vi "Reduce Funds.vi"(6 "wait for reply (T)":bool=TRUE, 8 "error in (no error)":errorcluster, 10 "Reduce Funds":i32) -> (0 "error out":errorcluster, 1 "timed out?":bool, 2 "Sucessful":bool, 3 "Remaining Balance":u32, 5 "Reply Payload":T1)   [LabVIEW 2020, in "Money.lvlib"]
doc: "Reduce Funds\n_____\nCreated using Delacor QMH Event Scripter 4.2.1.88."
uses:
  Money.lvlib
  Reduce Funds (Reply Payload)--cluster.ctl
  Reduce Funds Argument--cluster.ctl
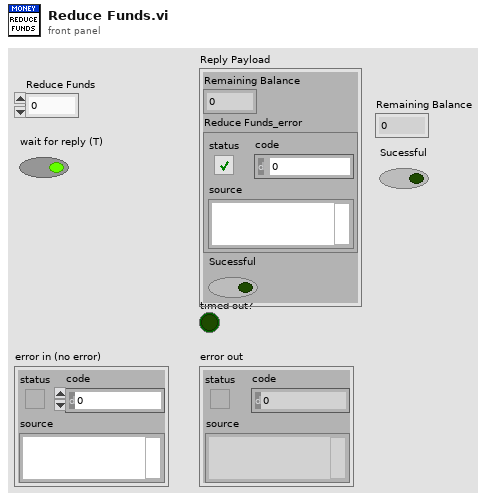
[diagram p1: front panel]
types:
  T1 = typedef "Money.lvlib/Reduce Funds (Reply Payload)--cluster.ctl" = cluster{"Remaining Balance":u32, "Reduce Funds_error":errorcluster, "Sucessful":bool}
  T2 = typedef "Money.lvlib/Reduce Funds Argument--cluster.ctl" = cluster{"Reduce Funds":i32, "Wait Notifier":refnum<notifier>, "wait for reply":bool}
  T3 = typedef "Money.lvlib/Request Events--cluster.ctl" = cluster{"Stop Module":refnum<user-event>, "Show Panel":refnum<user-event>, "Hide Panel":refnum<user-event>, "Get Module Execution Status":refnum<user-event>, "Show Diagram":refnum<user-event>, "Refund Money":refnum<user-event>, "Check Funds":refnum<user-event>, "Reduce Funds":refnum<user-event>, "Add to Balance":refnum<user-event>}
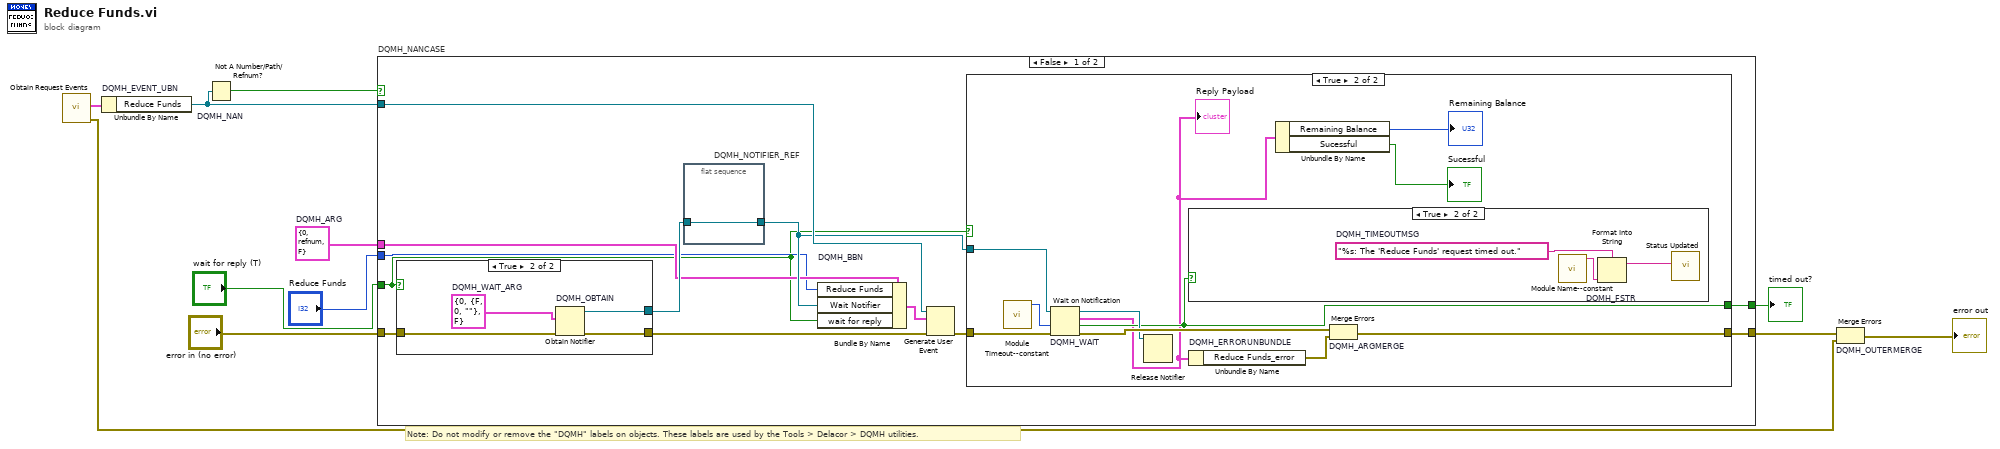
[diagram p0: block diagram]
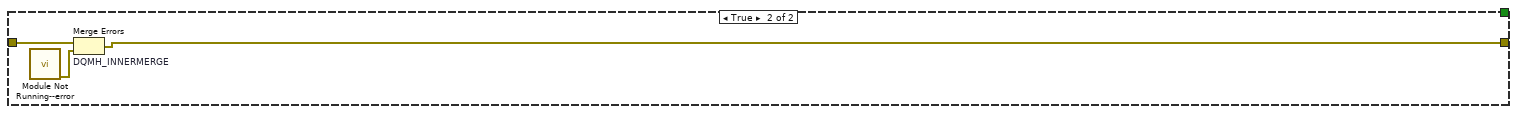
[diagram p5: hidden frame]
diagram:
  w5 = T2 {"Reduce Funds"=0, "Wait Notifier"=refnum, "wait for reply"=FALSE}  # DQMH_ARG
  # "Note: Do not modify or remove the \"DQMH\" labels on objects. These labels are used by the Tools > Delacor > DQMH utilities."
  n1 = call "Obtain Request Events.vi"() -> ("error out"=w2:errorcluster, "Money Request Events"=w1:T3)  [unwired: 10 in]
  n2 = Unbundle By Name "DQMH_EVENT_UBN"(w1) -> ("Reduce Funds"=w9:refnum<user-event>)
  n3 = Not A Number/Path/Refnum? "DQMH_NAN"(number/path/refnum=w9) -> (NaN/Path/Refnum?=w8:bool)
  n4 = case "DQMH_NANCASE" shown="False" w8 {
    tunnel: "error in (no error)" -> [w23 w47]
    tunnel: w9 -> [w21 _]
    tunnel: [w18 w46] -> w6
    tunnel: [w19 _] -> w7
    tunnel: w5 -> [w14 _]
    tunnel: "Reduce Funds" -> [w13 _]
    tunnel: "wait for reply (T)" -> [w12 _]
    frame False {
      n5 = case shown="True" w12 {
        tunnel: w23 -> [w40 w44]
        tunnel: [w40 w43] -> w20
        tunnel: [_ w41] -> w16
        frame False {
        }
        frame True {
          w42 = T1 {"Remaining Balance"=0, "Reduce Funds_error"={"status"=FALSE, "code"=0, "source"=""}, "Sucessful"=FALSE}  # DQMH_WAIT_ARG
          n6 = Obtain Notifier "DQMH_OBTAIN"(notification data type=w42, error in (no error)=w44) -> (notifier out=w41:refnum<notifier>, error out=w43:errorcluster)  [unwired: 2 in, 1 out]
        }
      }
      n7 = flat-sequence "DQMH_NOTIFIER_REF" {
        tunnel: w16 -> [w24]
        tunnel: [w24] -> w15
        frame #0 {
        }
      }
      n8 = Bundle By Name "DQMH_BBN"(cluster=w14, "Reduce Funds"=w13, "Wait Notifier"=w15, "wait for reply"=w12) -> (w17:T2)
      n9 = Generate User Event(user event=w21, event data cluster=w17, error in=w20) -> (error out=w22:errorcluster)  [unwired: 1 in, 1 out]
      n10 = case shown="True" w12 {
        tunnel: w22 -> [w25 w36]
        tunnel: w15 -> [_ w34]
        tunnel: [_ w32] -> w19
        tunnel: [w25 w31] -> w18
        frame False {
        }
        frame True {
          n11 = call "Module Timeout--constant.vi"() -> ("Module Timeout"=w29:i32)  [unwired: 11 in]
          n12 = Wait on Notification "DQMH_WAIT"(notifier=w34, timeout in ms (-1)=w29, error in (no error)=w36) -> (notifier out=w33:refnum<notifier>, notification=w28:T1, timed out?=w32:bool, error out=w35:errorcluster)  [unwired: 1 in]
          "Reply Payload" <- w28
          n13 = Release Notifier(notifier=w33) -> ()  [unwired: 2 in, 3 out]
          n14 = case shown="True" w32 {
            frame False {
            }
            frame True {
              w39 = "%s: The 'Reduce Funds' request timed out."  # DQMH_TIMEOUTMSG
              n15 = call "Module Name--constant.vi"() -> ("Module Name"=w38:string)  [unwired: 11 in]
              n16 = Format Into String "DQMH_FSTR"(format string=w39, w38) -> (resulting string=w37:string)  [unwired: 2 in, 1 out]
              n17 = call "Status Updated.vi"("Status"=w37) -> ()  [unwired: 10 in, 1 out]
            }
          }
          n18 = Unbundle By Name "DQMH_ERRORUNBUNDLE"(w28) -> ("Reduce Funds_error"=w30:errorcluster)
          n19 = Unbundle By Name(w28) -> ("Remaining Balance"=→"Remaining Balance":u32, "Sucessful"=→"Sucessful":bool)
          n20 = Merge Errors "DQMH_ARGMERGE"(w35, w30) -> (w31:errorcluster)
        }
      }
    }
    frame True {
      n21 = call "Module Not Running--error.vi"() -> ("error out"=w45:errorcluster)  [unwired: 11 in]
      n22 = Merge Errors "DQMH_INNERMERGE"(w47, w45) -> (w46:errorcluster)
    }
  }
  "timed out?" <- w7
  n23 = Merge Errors "DQMH_OUTERMERGE"(w6, w2) -> (→"error out":errorcluster)
